vi "1_4_Complex Exponential sequences.vi"() -> ()   [LabVIEW 2009]
panel:
  out "?":string
  in  "?":dbl=0.5 step=0.01
  in  "?":dbl=-0.088
  in  "?":dbl
  in  "|A|":dbl=1.0
  in  "stop":bool
  out "Imaginary Part":dbl[](graph)=[0.0, 0.43903915155573753, 0.7056727003162598, 0.7660497556521343, 0.6394908052507384, 0.38543785780666623, 0.083230232179901, -0.1894582053116094, -0.3743167315856812, -0.4427605489244637, -0.3977454027269251, -0.26799382213545847, -0.09719311881327887, 0.06852481596931222, 0.19164862563711044, 0.25057290703968055, 0.2420287442992139, 0.17888065078020504, 0.08454727907245604, -0.014118712225689386, -0.09359603793982631, -0.13859778707934778, -0.14427850374473905, -0.11566990915774603, -0.06492303342208003, -0.0073486756950955434, 0.04263401201989696, 0.07468887164265536, 0.0842946370562947, 0.07285231304370932, 0.04640536585069212, 0.013492620785861368, -0.017229529062466886, -0.039008375540429616, -0.04824961973603659, -0.04483904597879288, -0.03160731780711377, -0.013199976742925706, 0.0052899900058308155, 0.019572399925482164, 0.027022663760747336, 0.02702007308868562, 0.02076798383869277, 0.010721101143800099, -0.00018425500031964308, -0.00928706341099487, -0.014772684752946899, -0.015956008476704173, -0.013257637661164338, -0.00792815852143747]
  out "Real Part":dbl[](graph)=[1.0, 0.8036557762738299, 0.4531072301395103, 0.054324299150156054, -0.2926677979669427, -0.5159656669304553, -0.583881098656539, -0.5057807481124884, -0.3232940500334186, -0.0954774304958232, 0.11765822722039775, 0.26918251808023574, 0.3339898658196469, 0.31108446930371864, 0.2199197536013325, 0.09259853030188815, -0.03559397275797636, -0.13486539635670844, -0.1869209639498077, -0.18733967805525253, -0.14435794695775708, -0.07492177283755265, 0.0006385393372446925, 0.06385707769857628, 0.10210272812557364, 0.11055920074148853, 0.09207789663834817, 0.055280933035920486, 0.011635502315477497, -0.027657707288213446, -0.05421229392824669, -0.06394179561121159, -0.0573109821703587, -0.038493864043844854, -0.013809612089097601, 0.010085297588292281, 0.027791204365369547, 0.03621141191082349, 0.03489681693893383, 0.02572251578264631, 0.012078998531825196, -0.0021566504285900545, -0.013596074538170378, -0.02004452184131311, -0.020815878910335466, -0.016647906165497453, -0.009301801512359213, -0.0009896595350259417, 0.006209966821960285, 0.010811297697328213]
  in  "# of Samples":i32=50
  # "Exponential Sequences"
  # "Program Developed by Indranil Sinharoy"
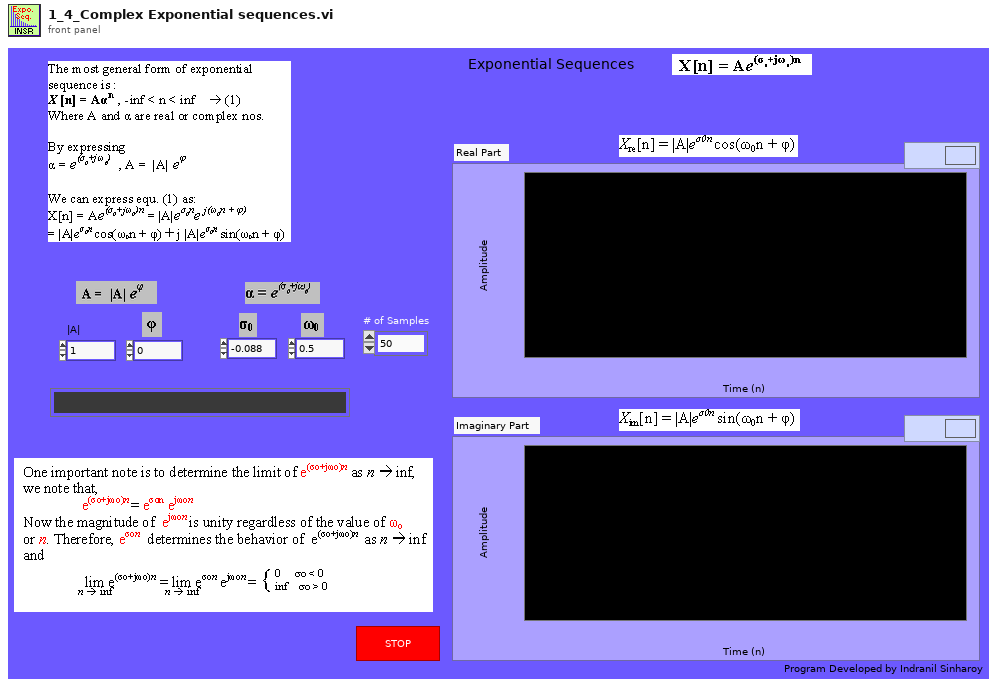
[diagram p1: front panel]
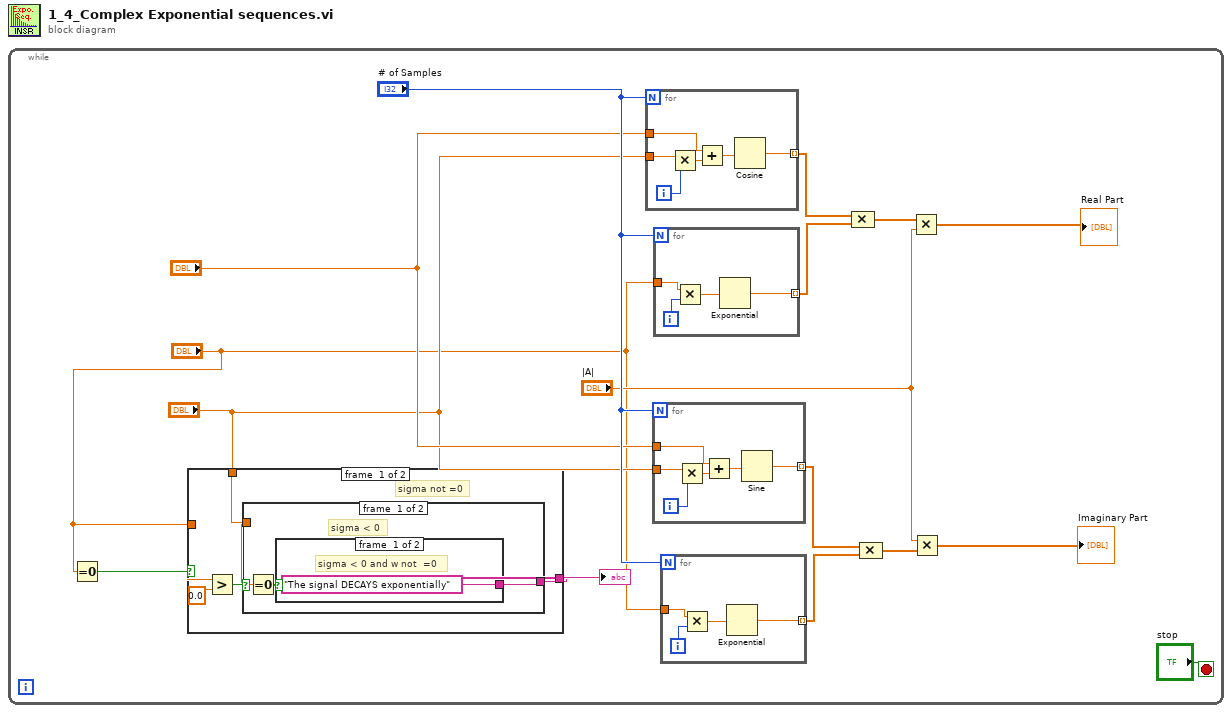
[diagram p0: block diagram]
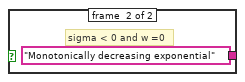
[diagram p2: hidden frame]
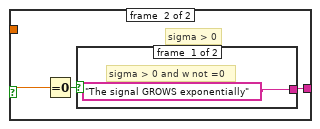
[diagram p3: hidden frame]
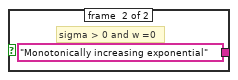
[diagram p4: hidden frame]
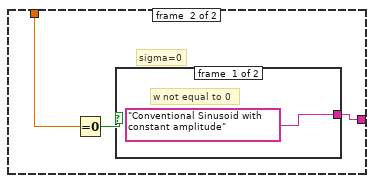
[diagram p5: hidden frame]
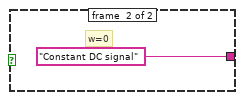
[diagram p6: hidden frame]
diagram:
  n1 = while {
    stop <- "stop" stop-if-true
    n2 = Equal To 0?(x="?") -> (x = 0?=w4:bool)
    n3 = case shown="True" w4 {
      tunnel: "?" -> [w18 w34]
      tunnel: [w17 w32] -> w2
      tunnel: "?" -> [w21 _]
      frame #0 {
        # "sigma not =0"
        n4 = Greater?(x=w21, y=0.0) -> (0:w19:bool)
        n5 = case shown="False" w19 {
          tunnel: w18 -> [w24 w28]
          tunnel: [w22 w27] -> w17
          frame #0 {
            # "sigma < 0"
            n6 = Equal To 0?(x=w24) -> (x = 0?=w23:bool)
            n7 = case shown="True" w23 {
              tunnel: ["The signal DECAYS exponentially" "Monotonically decreasing exponential"] -> w22
              frame #0 {
                # "sigma < 0 and w not  =0"
              }
              frame #1 {
                # "sigma < 0 and w =0"
              }
            }
          }
          frame #1 {
            # "sigma > 0"
            n8 = Equal To 0?(x=w28) -> (x = 0?=w29:bool)
            n9 = case shown="True" w29 {
              tunnel: ["The signal GROWS exponentially" "Monotonically increasing exponential"] -> w27
              frame #0 {
                # "sigma > 0 and w not =0"
              }
              frame #1 {
                # "sigma > 0 and w =0"
              }
            }
          }
        }
      }
      frame #1 {
        # "sigma=0"
        n10 = Equal To 0?(x=w34) -> (x = 0?=w33:bool)
        n11 = case shown="False" w33 {
          tunnel: ["Conventional Sinusoid with constant amplitude" "Constant DC signal"] -> w32
          frame #0 {
            # "w not equal to 0"
          }
          frame #1 {
            # "w=0"
          }
        }
      }
    }
    "?" <- w2
    n12 = for {
      N: "# of Samples" -> [_]
      tunnel: "?" -> [w53]
      tunnel: "?" -> [w55]
      tunnel: [w51] -> w16 mode=indexing
      i -> [w56]
      n13 = Multiply(x=w55, y=w56) -> (x*y=w54:dbl)
      n14 = Add(x=w53, y=w54) -> (x+y=w52:dbl)
      n15 = Cosine(x=w52) -> (cos(x)=w51:dbl)
    }
    n16 = for {
      N: "# of Samples" -> [_]
      tunnel: "?" -> [w43]
      tunnel: "?" -> [w45]
      tunnel: [w41] -> w10 mode=indexing
      i -> [w46]
      n17 = Multiply(x=w45, y=w46) -> (x*y=w44:dbl)
      n18 = Add(x=w43, y=w44) -> (x+y=w42:dbl)
      n19 = Sine(x=w42) -> (sin(x)=w41:dbl)
    }
    n20 = for {
      N: "# of Samples" -> [_]
      tunnel: "?" -> [w49]
      tunnel: [w47] -> w15 mode=indexing
      i -> [w50]
      n21 = Multiply(x=w49, y=w50) -> (x*y=w48:dbl)
      n22 = Exponential(1:w48) -> (0:w47:dbl)
    }
    n23 = for {
      N: "# of Samples" -> [_]
      tunnel: "?" -> [w39]
      tunnel: [w37] -> w9 mode=indexing
      i -> [w40]
      n24 = Multiply(x=w39, y=w40) -> (x*y=w38:dbl)
      n25 = Exponential(1:w38) -> (0:w37:dbl)
    }
    n26 = Compound Arithmetic op=MULTIPLY(w16, w15) -> (w14:dbl[])
    n27 = Compound Arithmetic op=MULTIPLY(w10, w9) -> (w8:dbl[])
    n28 = Multiply(x=w14, y="|A|") -> (x*y=→"Real Part":dbl[])
    n29 = Multiply(x="|A|", y=w8) -> (x*y=→"Imaginary Part":dbl[])
  }
